vi "Scanner-XYZ-Back.vi"(5 "加速度":dbl=900.0, 7 "最高速":dbl=1000.0, 8 "Error In":errorcluster, 10 "第一次位移":dbl[](array[numeric])=[0.0, 0.0, 0.0], 11 "X-Y-Z移動":dbl[](array[numeric])=[0.0, 0.0, 0.0]) -> (0 "Error Out":errorcluster, 1 "辨識結果(包含位置)":cluster{"讀取到時的位子":dbl, "辨識結果":string}[](array[cluster]), 2 "讀取到時的位子":dbl[](array[numeric]), 3 "辨識結果":string[](array[string]), 4 "辨識機率":i32[](array[numeric]))   [LabVIEW 2019]
uses:
  <vilib>/Platform/TimedLoop/XDataNode/timing_clust.ctl
  <vilib>/Platform/TimedLoop/XDataNode/nitl_modes.ctl
  <vilib>/Platform/TimedLoop/XDataNode/wakeup.ctl
  55a6ca66-6922-4a3f-b2ce-a8f2512fce50.vi
  Variable/Lock-PID.vi
  Variable/Position.vi
  <vilib>/platform/TimedLoop/XDataNode/XDataNode.xnode
  <vilib>/Platform/TimedLoop/XDataNode/XDNodeRunTimeDep.lvlib
panel:
  out "辨識機率":dbl[](array[slide]) scale=0.0..10.0
  out "三角形?":bool
  in  "Stop":bool
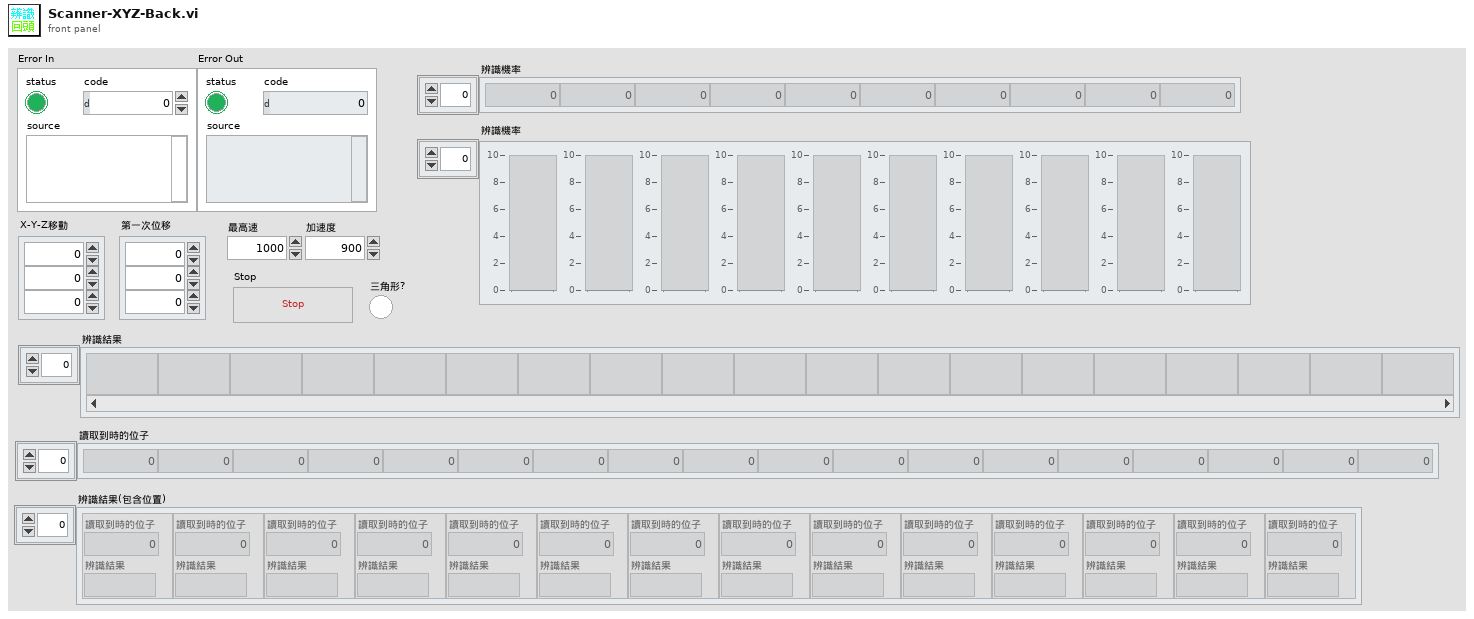
[diagram p1: front panel]
types:
  T1 = typedef "XDNodeRunTimeDep.lvlib/timing_clust.ctl" = cluster{"Expected End [f-1]":u64, "Actual End [f-1]":u64, "Finished Late? [f-1]":bool, "Expected End [i-1]":u64, "Actual End [i-1]":u64, "Finished Late? [i-1]":bool, "Expected Start [i]":u64, "Actual Start [i]":u64, "Expected Start [f]":u64, "Actual Start [f]":u64, "Source Name":string, "Structure Name":string, "Period":i64, "Deadline":i64, "Offset":i64, "Start":i64, "Priority":i32, "Timeout":i32, "Mode":T2, "Wakeup Reason":T3, "Error":errorcluster, "Source Type":string, "Secondary Source Type":string, "Global End Time":u64, "Global Start Time":u64, "Frame Duration":u64, "Iteration Duration":u64, "Assigned CPU":i32, "I/O Scan Engine Mode":u32}
  T2 = typedef "XDNodeRunTimeDep.lvlib/nitl_modes.ctl" = enum32{"No Change", "Process missed periods, maintain original phase", "Discard missed periods, maintain original phase", "Process missed periods, ignore original phase", "Discard missed periods, ignore original phase"}
  T3 = typedef "XDNodeRunTimeDep.lvlib/wakeup.ctl" = enum32{"Normal", "Aborted", "Asynchronous wakeup", "Timing source error", "Timed loop error", "Timeout"}
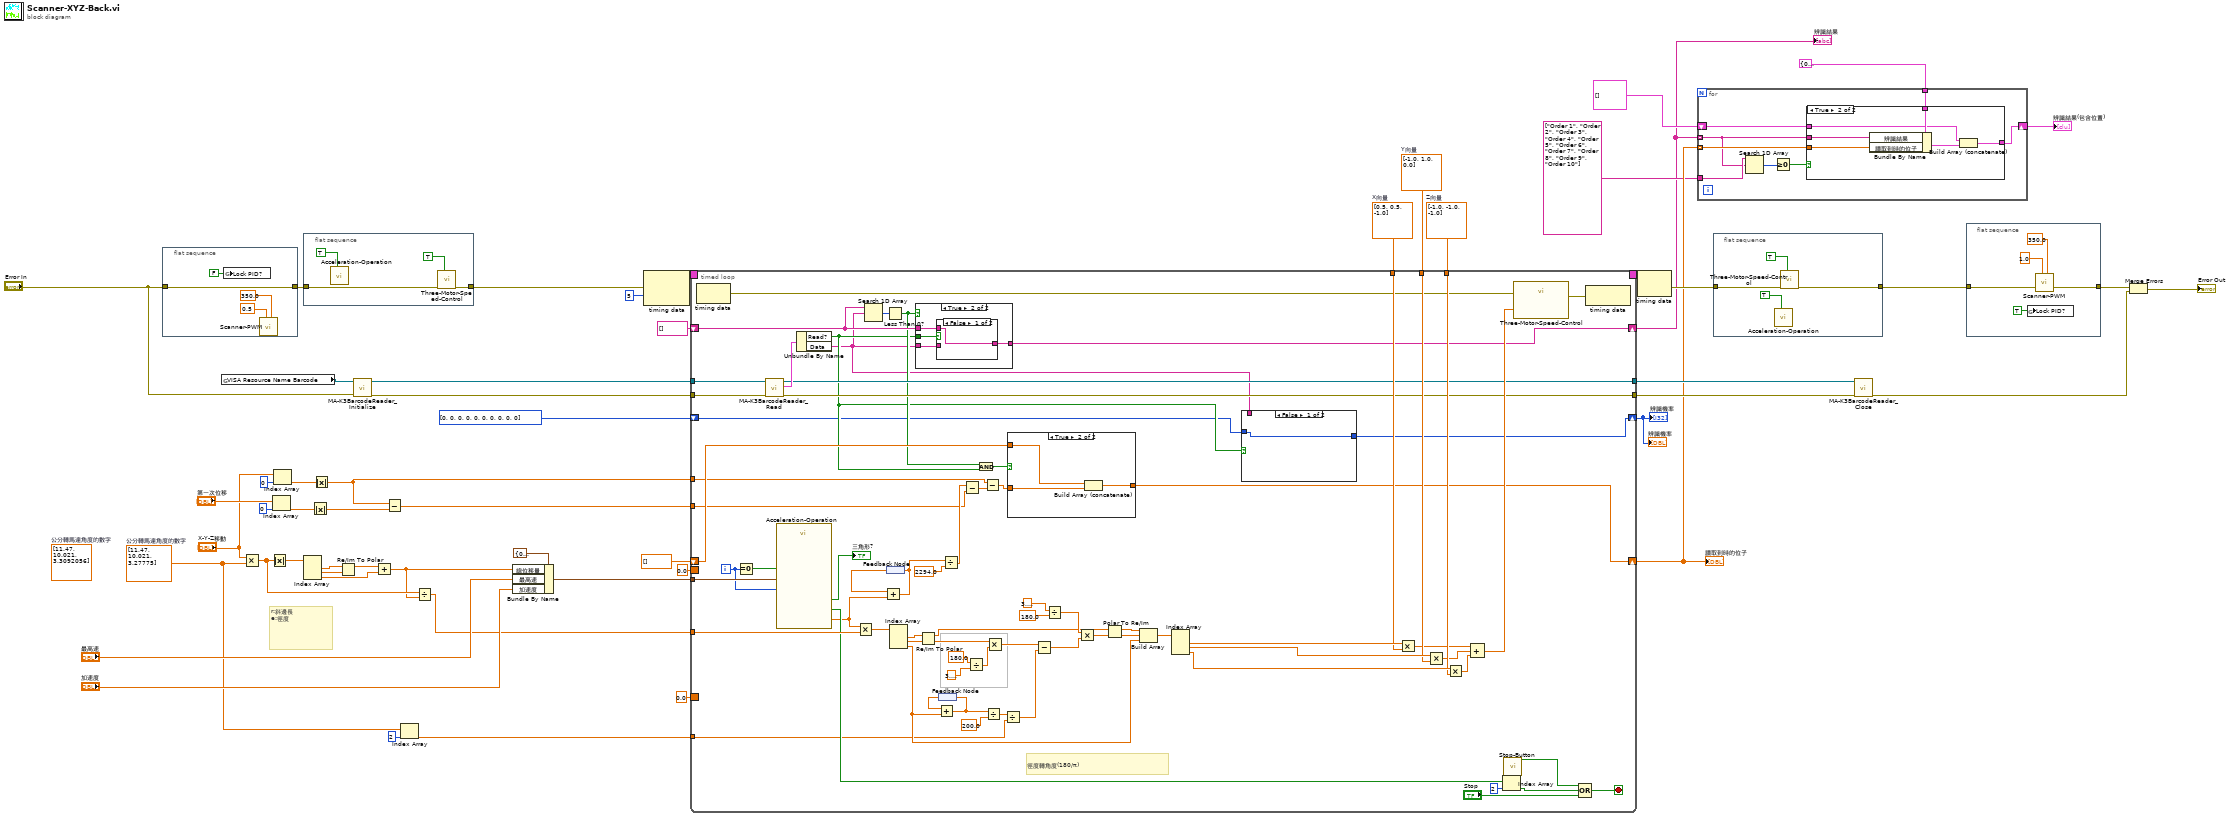
[diagram p0: block diagram]
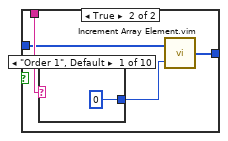
[diagram p3: hidden frame]
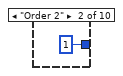
[diagram p4: hidden frame]
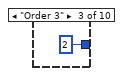
[diagram p5: hidden frame]
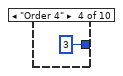
[diagram p6: hidden frame]
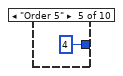
[diagram p7: hidden frame]
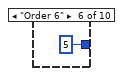
[diagram p8: hidden frame]
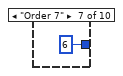
[diagram p9: hidden frame]
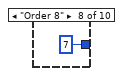
[diagram p10: hidden frame]
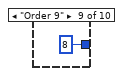
[diagram p11: hidden frame]
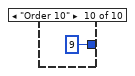
[diagram p12: hidden frame]
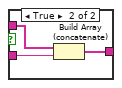
[diagram p14: hidden frame]
diagram:
  (unwired) dbl[] [11.47, 10.021, 3.3092056]  # 公分轉馬達角度的數字
  w36 = dbl[] [-1.0, -1.0, -1.0]  # Z向量
  w37 = dbl[] [-1.0, 1.0, 0.0]  # Y向量
  w38 = dbl[] [0.5, 0.5, -1.0]  # X向量
  w35 = dbl[] [11.47, 10.021, 3.27775]  # 公分轉馬達角度的數字
  # "r:斜邊長\ne:徑度"
  n1 = flat-sequence {
    tunnel: [w58] -> w31
    tunnel: "Error In" -> [w58]
    frame #0 {
      n2 = global write "Lock-PID.vi" "Lock PID?"(FALSE ("Lock PID?")) -> ()
      n3 = call "Scanner-PWM.vi"("Frequency [Hz]"=350.0, "Duty Cycle"=0.5) -> ()  [unwired: 9 in, 1 out]
    }
  }
  n4 = global read "Position.vi" "VISA Resource Name Barcode"() -> (w4:refnum<visa-resource-name>)
  n5 = Multiply(x="X-Y-Z移動", y=w35) -> (x*y=w42:dbl[])
  n6 = Absolute Value(x=w42) -> (abs(x)=w52:dbl[])
  n7 = Index Array(array="第一次位移", index=0) -> (element=w16:dbl)
  n8 = Index Array(array="X-Y-Z移動", index=0) -> (element=w14:dbl)
  n9 = Index Array(array=w52) -> (element #1=w49:dbl, element #2=w53:dbl, element #3=w50:dbl)  [unwired: 3 in]
  n10 = flat-sequence {
    tunnel: w31 -> [w62]
    tunnel: [w61] -> w41
    frame #0 {
      n11 = call "Acceleration-Operation.vi"("Reset"=TRUE) -> ()  [unwired: 8 in, 3 out]
      n12 = call "Three-Motor-Speed-Control.vi"("Reset"=TRUE, "Error In"=w62) -> ("Error Out"=w61:errorcluster)  [unwired: 9 in]
    }
  }
  n13 = Absolute Value(x=w16) -> (abs(x)=w11:dbl)
  n14 = Absolute Value(x=w14) -> (abs(x)=w9:dbl)
  n15 = Re/Im To Polar(2:w53, 3:w49) -> (1:w51:dbl)  [unwired: 1 out]
  n16 = call "MA-K3BarcodeReader_Initialize.vi"("Error In"="Error In", "掃碼機串口"=w4) -> ("Error Out"=w22:errorcluster, "VISA Resource"=w21:refnum<visa-resource-name>)  [unwired: 8 in]
  n17 = Add(x=w51, y=w50) -> (x+y=w30:dbl)
  n18 = Subtract(x=w9, y=w11) -> (x-y=w10:dbl)
  n19 = Index Array(array=w35, index=2) -> (element=w34:dbl)
  n20 = Divide(x=w42, y=w30) -> (x/y=w43:dbl[])
  n21 = Bundle By Name(cluster=cluster{"總位移量":dbl, "最高速":dbl, "加速度":dbl} {"總位移量"=0.0, "最高速"=0.0, "加速度"=0.0} ("計算設置"), "總位移量"=w30, "最高速"="最高速", "加速度"="加速度") -> (w44:cluster{"總位移量":dbl, "最高速":dbl, "加速度":dbl})
  n22 = node-c288(w41, i64 5 ("Period")) -> (w55:T1)
  n23 = timed-loop "Timed Loop" {
    timing: w55 -> [_]
    timing-out: [_] -> w54
    tunnel: w44 -> [w135]
    tunnel: w43 -> [w134]
    border: 0.0 -> [_]
    tunnel: w38 -> [w105]
    tunnel: w37 -> [w103]
    tunnel: w36 -> [w101]
    tunnel: w34 -> [w93]
    border: 0.0 -> [_]
    shift-right: [w86] -> w19
    shift-left: dbl[] [] -> [w85]
    tunnel: [w82] -> w25
    tunnel: [w81] -> w24
    shift-right: [w83] -> w3
    shift-left: string[] [] -> [w78]
    tunnel: w22 -> [w80]
    tunnel: w21 -> [w79]
    tunnel: w10 -> [w71]
    tunnel: w9 -> [w68]
    shift-right: [w64] -> w1
    shift-left: i32[] [0, 0, 0, 0, 0, 0, 0, 0, 0, 0] -> [w65]
    i -> [w132]
    stop <- w131 stop-if-true
    # "徑度轉角度(180/π)"
    n24 = node-c288() -> (w96:errorcluster)  [unwired: 1 in]
    n25 = Equal To 0?(x=w132) -> (x = 0?=w133:bool)
    n26 = call "MA-K3BarcodeReader_Read.vi"("error in (no error)"=w80, "VISA Reference"=w79) -> ("error out"=w82:errorcluster, "Result"=w84:cluster{"Read?":bool, "Data":string}, "VISA Reference"=w81:refnum<visa-resource-name>)  [unwired: 7 in]
    n27 = call "Acceleration-Operation.vi"("Reset"=w133, "迴圈( I )"=w132, "計算設置"=w135) -> ("完成?"=w130:bool[], "速度"=w73:dbl, "三角形?"=→"三角形?":bool)  [unwired: 6 in]
    n28 = Unbundle By Name(w84) -> ("Read?"=w67:bool, "Data"=w66:string)
    n29 = Multiply(x=w73, y=w134) -> (x*y=w127:dbl[])
    n30 = Search 1D Array(1D array=w78, element=w66) -> (index of element=w77:i32)  [unwired: 1 in]
    n31 = Less Than 0?(x=w77) -> (x < 0?=w75:bool)
    n32 = feedback #1() -> (w89:dbl)
    n33 = Add(x=w89, y=w73) -> (x+y=w88:dbl)
    n34 = feedback-in #1(w88) -> ()
    n35 = Index Array(array=w127) -> (element #1=w126:dbl, element #2=w125:dbl, element #3=w108:dbl)  [unwired: 3 in]
    n36 = case shown="True" w75 {
      tunnel: w66 -> [_ w155]
      tunnel: w67 -> [_ w154]
      tunnel: [w151 w153] -> w83
      tunnel: w78 -> [w151 w152]
      frame False {
      }
      frame True {
        n37 = case shown="False" w154 {
          tunnel: w155 -> [_ w159]
          tunnel: [w156 w158] -> w153
          tunnel: w152 -> [w156 w157]
          frame False {
          }
          frame True {
            n38 = Build Array (concatenate)(w157, w159) -> (w158:string[])
          }
        }
      }
    }
    n39 = Re/Im To Polar(2:w125, 3:w126) -> (0:w124:dbl, 1:w111:dbl)
    n40 = feedback #2() -> (w120:dbl)
    n41 = Add(x=w120, y=w108) -> (x+y=w119:dbl)
    n42 = feedback-in #2(w119) -> ()
    n43 = Divide(x=w88, y=2294.0) -> (x/y=w72:dbl)
    n44 = Subtract(x=w72, y=w71) -> (x-y=w70:dbl)
    n45 = Divide(x=180.0, y=3.141592653589793) -> (x/y=w121:dbl)
    n46 = And(x=w75, y=w67) -> (x .and. y?=w76:bool)
    n47 = Subtract(x=w68, y=w70) -> (x-y=w69:dbl)
    n48 = Divide(x=w119, y=200.0) -> (x/y=w95:dbl)
    n49 = Multiply(x=w124, y=w121) -> (x*y=w117:dbl)
    n50 = Divide(x=w95, y=w93) -> (x/y=w94:dbl)
    n51 = case shown="True" w76 {
      tunnel: w69 -> [_ w163]
      tunnel: [w160 w162] -> w86
      tunnel: w85 -> [w160 w161]
      frame False {
      }
      frame True {
        n52 = Build Array (concatenate)(w161, w163) -> (w162:dbl[])
      }
    }
    n53 = Subtract(x=w117, y=w94) -> (x-y=w113:dbl)
    n54 = Divide(x=3.141592653589793, y=180.0 ("x")) -> (x/y=w114:dbl)
    n55 = Multiply(x=w114, y=w113) -> (x*y=w112:dbl)
    n56 = Polar To Re/Im(2:w112, 3:w111) -> (0:w109:dbl, 1:w110:dbl)
    n57 = Build Array(w110, w109, w108) -> (w107:dbl[])
    n58 = Index Array(array=w107) -> (element #1=w106:dbl, element #2=w104:dbl, element #3=w102:dbl)  [unwired: 3 in]
    n59 = case shown="False" w67 {
      tunnel: w66 -> [_ w140]
      tunnel: w65 -> [w136 w138]
      tunnel: [w136 w137] -> w64
      frame False {
      }
      frame True {
        n60 = case shown="\"Order 1\", Default" w140 {
          tunnel: [0 1 2 3 4 5 6 7 8 9] -> w139
          frame "Order 1", Default {
          }
          frame "Order 2" {
          }
          frame "Order 3" {
          }
          frame "Order 4" {
          }
          frame "Order 5" {
          }
          frame "Order 6" {
          }
          frame "Order 7" {
          }
          frame "Order 8" {
          }
          frame "Order 9" {
          }
          frame "Order 10" {
          }
        }
        n61 = call "Increment Array Element.vim"("index"=w139, "array in"=w138) -> ("array out"=w137:i32[])
      }
    }
    n62 = Multiply(x=w106, y=w105) -> (x*y=w100:dbl[])
    n63 = Multiply(x=w104, y=w103) -> (x*y=w99:dbl[])
    n64 = Multiply(x=w102, y=w101) -> (x*y=w98:dbl[])
    n65 = Compound Arithmetic op=ADD(w100, w99, w98) -> (w90:dbl[])
    n66 = Index Array(array=w130, index=2) -> (element=w91:bool)
    n67 = call "Stop-Button.vi"() -> ("顯示按下?"=w92:bool)  [unwired: 10 in, 1 out]
    n68 = call "Three-Motor-Speed-Control.vi"("Error In"=w96, "速度(秒/度)"=w90) -> ("Error Out"=w97:errorcluster)  [unwired: 9 in]
    n69 = Compound Arithmetic op=OR(w92, w91, "Stop") -> (w131:bool)
    n70 = node-c288(w97) -> ()  [unwired: 1 out]
  }
  "辨識結果" <- w3
  "讀取到時的位子" <- w19
  "辨識機率" <- w1
  "辨識機率" <- w1
  n71 = node-c288(w54) -> (w40:errorcluster)
  n72 = for {
    tunnel: w3 -> [w172] mode=indexing
    tunnel: cluster{"讀取到時的位子":dbl, "辨識結果":string} {"讀取到時的位子"=0.0, "辨識結果"=""} ("input cluster") -> [w176]
    tunnel: w19 -> [w175] mode=indexing
    tunnel: string[] ["Order 1", "Order 2", "Order 3", "Order 4", "Order 5", "Order 6", "Order 7", "Order 8", "Order 9", "Order 10"] -> [w173]
    shift-right: [w174] -> w6
    shift-left: cluster{"讀取到時的位子":dbl, "辨識結果":string}[] [] -> [w169]
    n73 = Search 1D Array(1D array=w173, element=w172) -> (index of element=w171:i32)  [unwired: 1 in]
    n74 = Greater Or Equal To 0?(x=w171) -> (x >= 0?=w170:bool)
    n75 = case shown="True" w170 {
      tunnel: w172 -> [_ w183]
      tunnel: w176 -> [_ w182]
      tunnel: w175 -> [_ w181]
      tunnel: [w177 w178] -> w174
      tunnel: w169 -> [w177 w179]
      frame False {
      }
      frame True {
        n76 = Bundle By Name(cluster=w182, "辨識結果"=w183, "讀取到時的位子"=w181) -> (w180:cluster{"讀取到時的位子":dbl, "辨識結果":string})
        n77 = Build Array (concatenate)(w179, w180) -> (w178:cluster{"讀取到時的位子":dbl, "辨識結果":string}[])
      }
    }
  }
  "辨識結果(包含位置)" <- w6
  n78 = flat-sequence {
    tunnel: w40 -> [w186]
    tunnel: [w185] -> w32
    frame #0 {
      n79 = call "Acceleration-Operation.vi"("Reset"=TRUE) -> ()  [unwired: 8 in, 3 out]
      n80 = call "Three-Motor-Speed-Control.vi"("Reset"=TRUE, "Error In"=w186) -> ("Error Out"=w185:errorcluster)  [unwired: 9 in]
    }
  }
  n81 = call "MA-K3BarcodeReader_Close.vi"("Error In"=w25, "VISA Resource"=w24) -> ("Error Out"=w18:errorcluster)  [unwired: 9 in]
  n82 = flat-sequence {
    tunnel: [w190] -> w29
    tunnel: w32 -> [w190]
    frame #0 {
      n83 = global write "Lock-PID.vi" "Lock PID?"(TRUE ("Lock PID?")) -> ()
      n84 = call "Scanner-PWM.vi"("Frequency [Hz]"=350.0, "Duty Cycle"=1.0) -> ()  [unwired: 9 in, 1 out]
    }
  }
  n85 = Merge Errors(w29, w18) -> (→"Error Out":errorcluster)
